vi "Write TestStatus.vi"(10 "TestStatus":T1={"activeCycle"=0, "activeProfileStep"=0, "demandedCycles"=0, "demandedProfileSteps"=0, "temperatureSetpoint"=275.15, "pgaGainCoefficient"=0} {"temperatureSetpoint" min=271.15 max=275.15 format="%.1f"; "pgaGainCoefficient" min=1; "demandedProfileSteps" min=1; "demandedCycles" min=1; "activeProfileStep" min=1; "activeCycle" min=1}, 11 "Logger in":refnum<class "TestDataLog.lvclass">) -> (3 "Logger out":refnum<class "TestDataLog.lvclass">)   [LabVIEW 2013, in "TestDataLog.lvclass"]
uses:
  TestDataLog.lvclass
  Typedefs/TestStatus.ctl
  TestDataLog.lvclass/TestDataLog.ctl
  Typedefs/AITDTTypedefs.lvlib
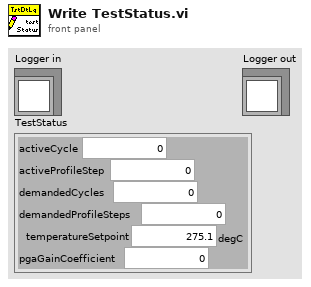
[diagram p1: front panel]
types:
  T1 = typedef "AITDTTypedefs.lvlib/TestStatus.ctl" = cluster{"activeCycle":u32, "activeProfileStep":u32, "demandedCycles":u32, "demandedProfileSteps":u32, "temperatureSetpoint":dbl[unit], "pgaGainCoefficient":u16}
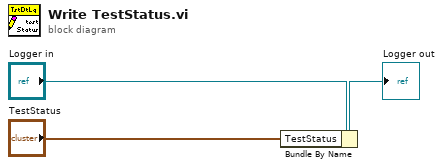
[diagram p0: block diagram]
diagram:
  n1 = Bundle By Name(cluster="Logger in", "TestStatus"="TestStatus") -> (→"Logger out":refnum<class "TestDataLog.lvclass">)
